vi "getId.vi"(8 "error in (no error)":errorcluster, 11 "CompoundShape in":refnum<class "CompoundShape.lvclass">) -> (0 "error out":errorcluster, 2 "id":i32, 3 "CompoundShape out":refnum<class "CompoundShape.lvclass">)   [LabVIEW 2017, in "CompoundShape.lvclass"]
uses:
  CompoundShape.lvclass
  CompoundShape.lvclass/CompoundShape.ctl
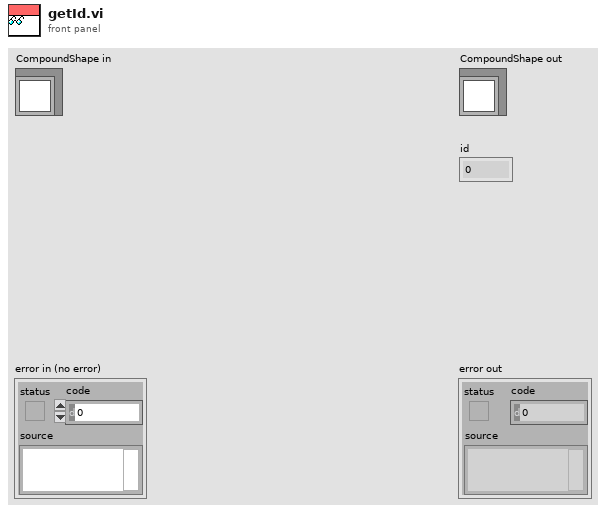
[diagram p1: front panel]
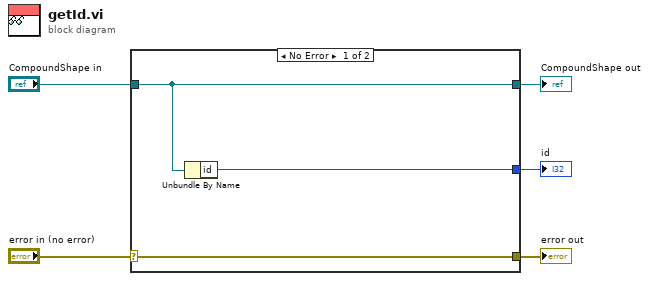
[diagram p0: block diagram]
diagram:
  n1 = case shown="No Error" "error in (no error)" {
    selector: "error in (no error)" -> [w8 w9]
    tunnel: [w8 w9] -> w4
    tunnel: [w7 w10] -> w2
    tunnel: "CompoundShape in" -> [w7 w10]
    tunnel: [w6 _] -> w1
    frame No Error {
      n2 = Unbundle By Name(w7) -> ("id"=w6:i32)
    }
    frame Error {
    }
  }
  "error out" <- w4
  "CompoundShape out" <- w2
  "id" <- w1
